vi "SimpleTrafficLights.vi"() -> ()   [LabVIEW 2015]
panel:
  in  "stop":bool
  out "Boolean 3":bool
  out "Boolean 2":bool
  out "Boolean":bool
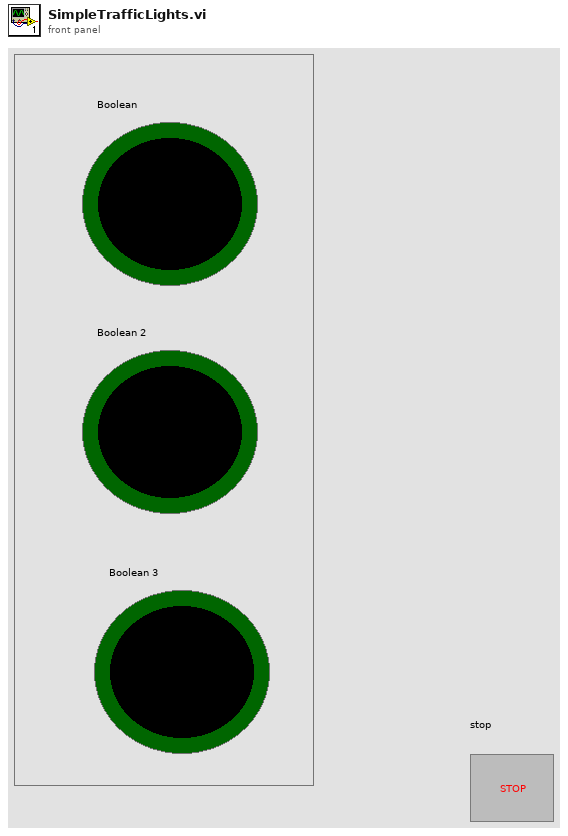
[diagram p1: front panel]
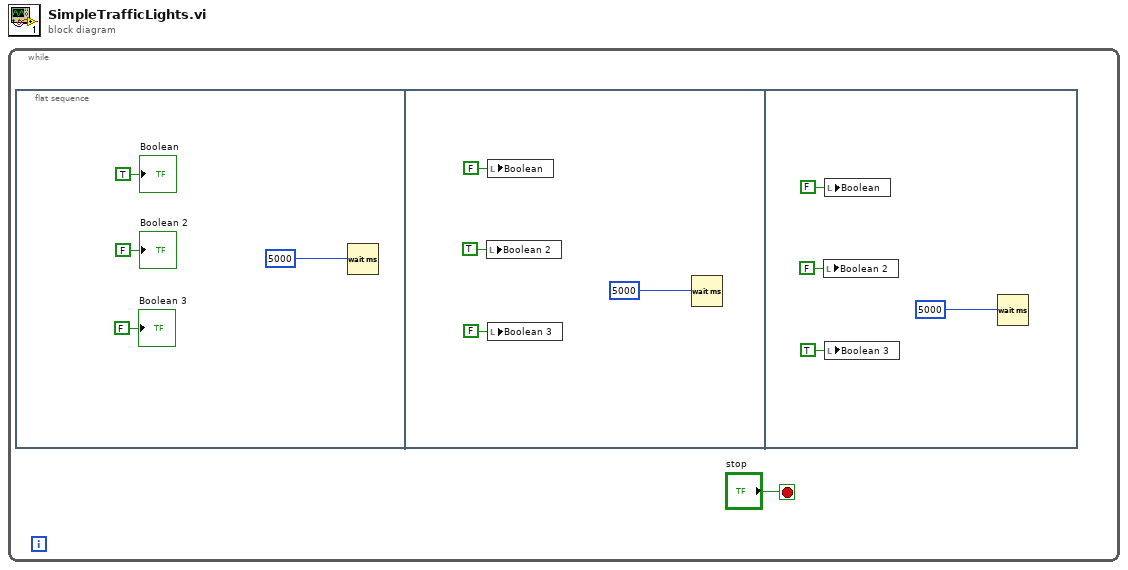
[diagram p0: block diagram]
diagram:
  n1 = while {
    stop <- "stop" stop-if-true
    n2 = flat-sequence {
      frame #0 {
        n3 = Wait (ms)(milliseconds to wait=u32 5000 ("millisecond timer value")) -> ()  [unwired: 1 out]
        "Boolean 2" <- FALSE ("Boolean 2")
        "Boolean" <- TRUE ("Boolean")
        "Boolean 3" <- FALSE ("Boolean 3")
      }
      frame #1 {
        n4 = local write "Boolean 2"(TRUE ("Boolean 2")) -> ()
        n5 = local write "Boolean"(FALSE ("Boolean")) -> ()
        n6 = local write "Boolean 3"(FALSE ("Boolean 3")) -> ()
        n7 = Wait (ms)(milliseconds to wait=u32 5000 ("millisecond timer value")) -> ()  [unwired: 1 out]
      }
      frame #2 {
        n8 = local write "Boolean 2"(FALSE ("Boolean 2")) -> ()
        n9 = local write "Boolean"(FALSE ("Boolean")) -> ()
        n10 = local write "Boolean 3"(TRUE ("Boolean 3")) -> ()
        n11 = Wait (ms)(milliseconds to wait=u32 5000 ("millisecond timer value")) -> ()  [unwired: 1 out]
      }
    }
  }
